vi "Transition Type.vi"(11 "Transition Config in":refnum<class "Transition Config.lvclass">) -> (2 "Transition Type":string)   [LabVIEW 2020, in "VolatusSeqConfig.lvlib" / "Transition Config.lvclass"]
uses:
  Transition Config.lvclass
  Transition Config.lvclass/Transition Config.ctl
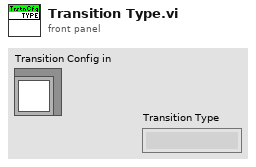
[diagram p1: front panel]
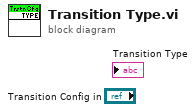
[diagram p0: block diagram]
diagram:
